vi "GEM_BANK_BuildHeader.vi"(0 "LVBANK in":refnum<class "GEM_BANK.lvclass">, 5 "GEM BANK cluster":T1, 11 "error in (no error)":errorcluster) -> (4 "LVBANK out":refnum<class "GEM_BANK.lvclass">, 15 "error out":errorcluster)   [LabVIEW 2018, in "feGEM DataPacker.lvlib" / "GEM_BANK.lvclass"]
uses:
  GEM_BANK.lvclass
  GEM_BANK_CLUSTER_typedef.ctl
  GEM_DATA_cluster_typedef.ctl
  GEM_BANK.lvclass/GEM_BANK.ctl
  feGEM DataPacker.lvlib
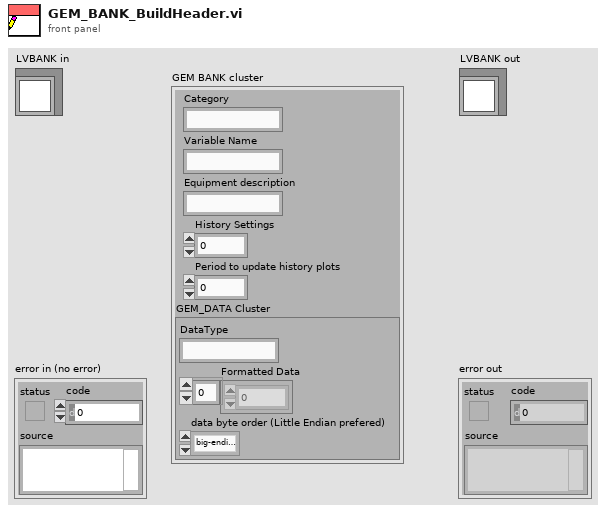
[diagram p1: front panel]
types:
  T1 = typedef "feGEM DataPacker.lvlib/GEM_BANK_CLUSTER_typedef.ctl" = cluster{"Category":string, "Variable Name":string, "Equipment description":string, "History Settings":u16, "Period to update history plots":u16, "GEM_DATA Cluster":T2}
  T2 = typedef "feGEM DataPacker.lvlib/GEM_DATA_cluster_typedef.ctl" = cluster{"DataType":string, "Formatted Data":u8[], "data byte order (Little Endian prefered)":enum16{"big-endian, network order", "native, host order", "little-endian"}}
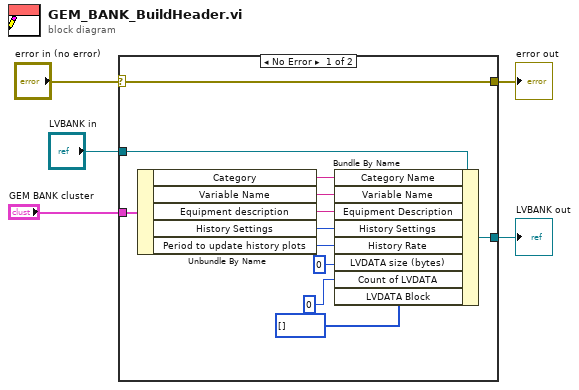
[diagram p0: block diagram]
diagram:
  n1 = case shown="No Error" "error in (no error)" {
    selector: "error in (no error)" -> [w17 w18]
    tunnel: [w17 w18] -> w4
    tunnel: [w15 w19] -> w2
    tunnel: "LVBANK in" -> [w16 w19]
    tunnel: "GEM BANK cluster" -> [w14 _]
    frame No Error {
      n2 = Unbundle By Name(w14) -> ("Category"=w13:string, "Variable Name"=w12:string, "Equipment description"=w11:string, "History Settings"=w9:u16, "Period to update history plots"=w8:u16)
      n3 = Bundle By Name(cluster=w16, "Category Name"=w13, "Variable Name"=w12, "Equipment Description"=w11, "History Settings"=w9, "History Rate"=w8, "LVDATA size (bytes)"=u32 0, "Count of LVDATA"=0, "LVDATA Block"=u8[] []) -> (w15:refnum<class "GEM_BANK.lvclass">)
    }
    frame Error {
    }
  }
  "error out" <- w4
  "LVBANK out" <- w2
